vi "Tab Control - Get Tab Control Real Value.vi"(8 "error in (no error)":errorcluster, 10 "control label":string, 11 "page ref":refnum<vi>) -> (0 "error out":errorcluster, 3 "value":dbl)   [LabVIEW 2020]
doc: "Get real valued control by name from provided page."
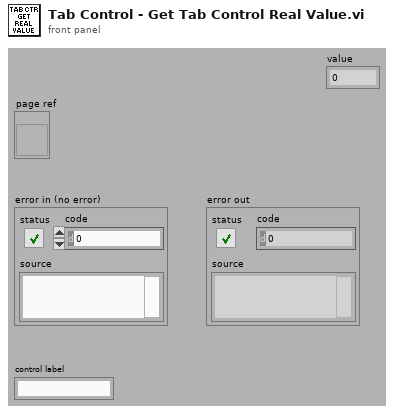
[diagram p1: front panel]
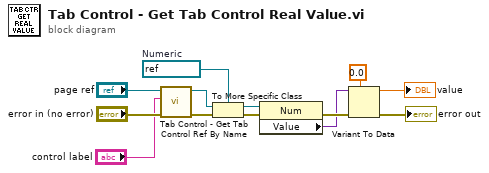
[diagram p0: block diagram]
diagram:
  w6 = refnum<vi> refnum  # Numeric
  n1 = call "Tab Control - Get Tab Control Ref By Name.vi"("error in (no error)"="error in (no error)", "control label"="control label", "page ref"="page ref") -> ("error out"=w10:errorcluster, "control ref out"=w8:refnum<vi>)  [unwired: 7 in]
  n2 = To More Specific Class(target class=w6, reference=w8, error in=w10) -> (specific class reference=w7:refnum<vi>, error out=w9:errorcluster)
  n3 = property class="Num"(reference=w7, error in=w9) -> (error out=w5:errorcluster, "Value"=w4:variant)  [unwired: 1 out]
  n4 = Variant To Data(error in=w5, type=0.0, Variant=w4) -> (data=→"value":dbl, error out=→"error out":errorcluster)
